vi "GetWave.vi"(2 "error in (no error)":errorcluster) -> (0 "error out":errorcluster, 1 "Present Wavelength":dbl format="%.4f")   [LabVIEW 2017]
doc: "Returns the present wavelength position of the monochromator.\nPresent Wavelength is presented in the global Wavelength Units."
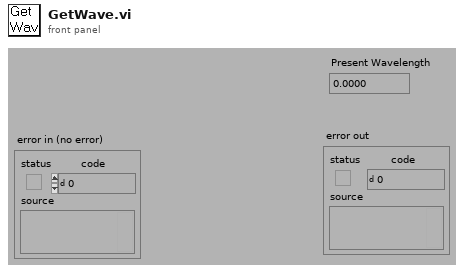
[diagram p1: front panel]
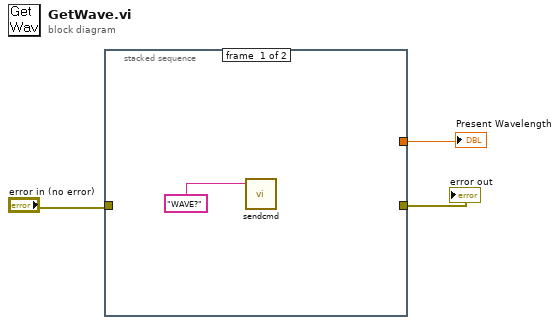
[diagram p0: block diagram]
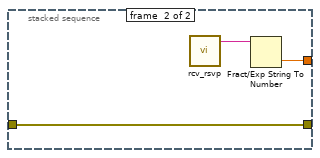
[diagram p2: hidden frame]
diagram:
  n1 = stacked-sequence {
    tunnel: "error in (no error)" -> [_ w5]
    tunnel: [_ w7] -> w2
    tunnel: [_ w5] -> w1
    frame #0 {
      n2 = call "sendcmd.vi"("command in"="WAVE?") -> ()  [unwired: 2 in, 1 out]
    }
    frame #1 {
      n3 = call "rcv_rsvp.vi"() -> ("response string"=w6:string)  [unwired: 2 in, 1 out]
      n4 = Fract/Exp String To Number(string=w6) -> (number=w7:dbl)  [unwired: 3 in, 1 out]
    }
  }
  "error out" <- w1
  "Present Wavelength" <- w2
